vi "Radau5_Error Tolerance.vi"(9 "Relative Tolerance":dbl[](array[numeric]), 10 "Absolute Tolerance":dbl[](array[numeric]), 11 "Y in":dbl[](array[numeric])) -> (3 "Error tolerance":dbl[](array[numeric]))   [LabVIEW 2017, in "NI_DAE.lvlib"]
uses:
  <vilib>/gmath/NI_DAE.lvlib
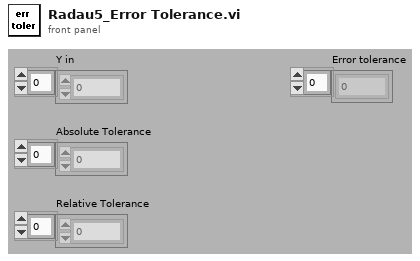
[diagram p1: front panel]
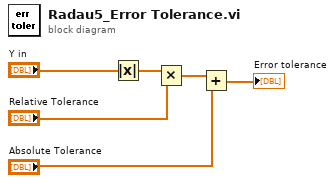
[diagram p0: block diagram]
diagram:
  n1 = Absolute Value(x="Y in") -> (abs(x)=w5:dbl[])
  n2 = Multiply(x=w5, y="Relative Tolerance") -> (x*y=w4:dbl[])
  n3 = Add(x=w4, y="Absolute Tolerance") -> (x+y=→"Error tolerance":dbl[])
